vi "PH_gentec_M-Link.set i Attr.vi"(0 "i ref in":refnum<vi>, 5 "error in":errorcluster) -> (14 "i ref out":refnum<vi>, 16 "i Attributes":T1 {"Current Head Settings"."Waveform Averages" items=["None", "2", "4", "8", "16", "32", "64", "128"]; "Current Head Settings"."Trigger Source" items=["Internal", "External"]; "Current Head Settings"."Trigger Polarity" items=["Falling Edge", "Rising Edge"]; "Current Head Settings"."Measurement Mode" items=["other Mode", "Energymode"]; "Wanted Head Settings"."Waveform Averages" items=["None", "2", "4", "8", "16", "32", "64", "128"]; "Wanted Head Settings"."Trigger Source" items=["Internal", "External"]; "Wanted Head Settings"."Trigger Polarity" items=["Falling Edge", "Rising Edge"]; "Wanted Head Settings"."Measurement Mode" items=["other Mode", "Energymode"]}, 19 "error out":errorcluster)   [LabVIEW 2014, in "PH_gentec_M-Link.lvlib"]
doc: "This VI reads the DB entries and sets several attributes and GUI element settings."
uses:
  PH_gentec_M-Link.lvlib
  PH_gentec_M-Link.i attribute.ctl
  PH_gentec_M-Link.Head Settings.ctl
  instr.lib/Gentec-M-Link/Driver/Type Defs/gentec-M-Link.Measurement Mode.ctl
  instr.lib/Gentec-M-Link/Driver/Type Defs/gentec-M-Link.Trigger Polarity.ctl
  instr.lib/Gentec-M-Link/Driver/Type Defs/gentec-M-Link.Trigger Source.ctl
  instr.lib/Gentec-M-Link/Driver/Type Defs/gentec-M-Link.Waveform Averages.ctl
  instr.lib/Gentec-M-Link/gentec-M-Link - Driver.lvlib
  PH_Basics/PH_Common/PH_Common.lvlib
  CS_Core/CSSystem/CSSystemLib/CSSystemLib.lvlib
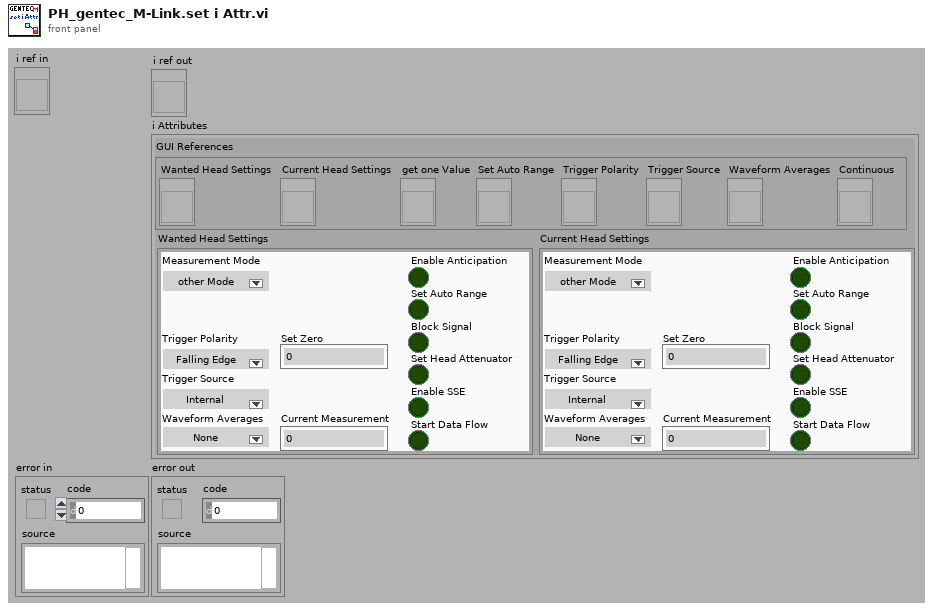
[diagram p1: front panel]
types:
  T1 = typedef "PH_gentec_M-Link.lvlib/PH_gentec_M-Link.i attribute.ctl" = cluster{"GUI References":cluster{"Wanted Head Settings":refnum<vi>, "Current Head Settings":refnum<vi>, "Set Auto Range":refnum<vi>, "Trigger Polarity":refnum<vi>, "Trigger Source":refnum<vi>, "Waveform Averages":refnum<vi>, "Continuous":refnum<vi>, "get one Value":refnum<vi>}, "Wanted Head Settings":T2, "Current Head Settings":T2}
  T2 = typedef "PH_gentec_M-Link.lvlib/PH_gentec_M-Link.Head Settings.ctl" = cluster{"Measurement Mode":T3, "Enable Anticipation":bool, "Set Auto Range":bool, "Block Signal":bool, "Set Head Attenuator":bool, "Enable SSE":bool, "Trigger Polarity":T4, "Trigger Source":T5, "Waveform Averages":T6, "Set Zero":i32, "Current Measurement":i32, "Start Data Flow":bool}
  T3 = typedef "gentec-M-Link - Driver.lvlib/gentec-M-Link.Measurement Mode.ctl" = u16
  T4 = typedef "gentec-M-Link - Driver.lvlib/gentec-M-Link.Trigger Polarity.ctl" = u16
  T5 = typedef "gentec-M-Link - Driver.lvlib/gentec-M-Link.Trigger Source.ctl" = u16
  T6 = typedef "gentec-M-Link - Driver.lvlib/gentec-M-Link.Waveform Averages.ctl" = u16
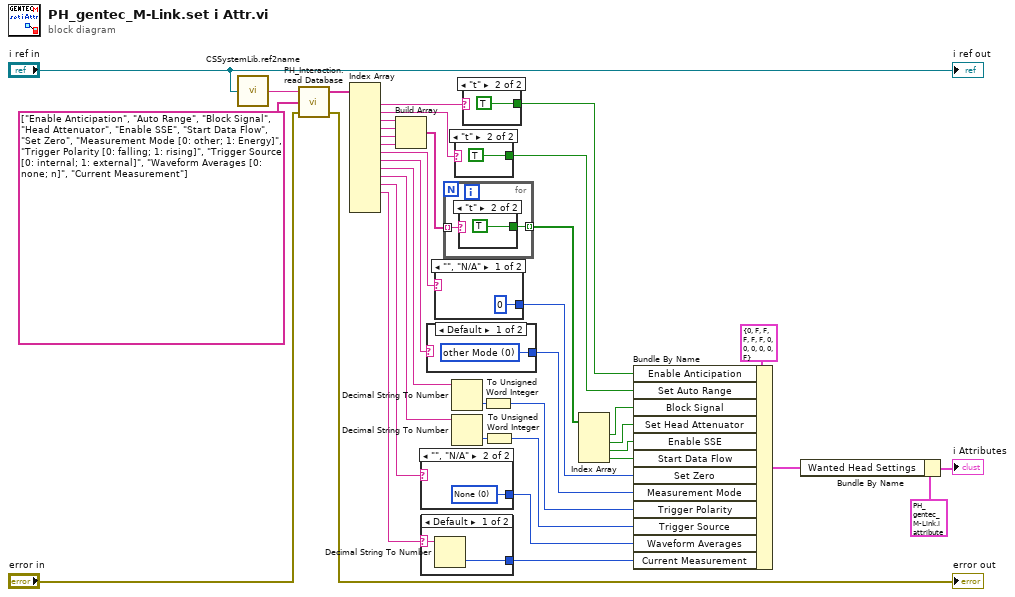
[diagram p0: block diagram]
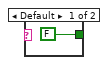
[diagram p2: hidden frame]
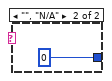
[diagram p3: hidden frame]
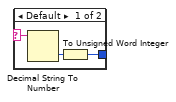
[diagram p4: hidden frame]
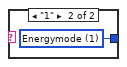
[diagram p5: hidden frame]
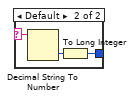
[diagram p6: hidden frame]
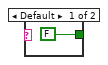
[diagram p7: hidden frame]
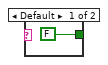
[diagram p8: hidden frame]
diagram:
  n1 = call "CSSystemLib.ref2name.vi"("obj refnum"="i ref in") -> ("name"=w19:string)
  n2 = call "PH_Interaction.read Database.vi"("error in (no error)"="error in", "Strings to search for"=string[] ["Enable Anticipation", "Auto Range", "Block Signal", "Head Attenuator", "Enable SSE", "Start Data Flow", "Set Zero", "Measurement Mode [0: other; 1: Energy]", "Trigger Polarity [0: falling; 1: rising]", "Trigger Source [0: internal; 1: external]", "Waveform Averages [0: none; n]", "Current Measurement"], "DB Entry to read"=w19) -> ("error out"=→"error out":errorcluster, "Values"=w17:string[])  [unwired: 1 in]
  n3 = Index Array(array=w17) -> (element #1=w12:string, element #2=w11:string, element #3=w10:string, element #4=w9:string, element #5=w8:string, element #6=w7:string, element #7=w6:string, element #8=w5:string, element #9=w4:string, element #10=w3:string, element #11=w2:string, element #12=w1:string)  [unwired: 14 in, 2 out]
  n4 = Build Array(w10, w9, w8, w7) -> (w33:string[])
  n5 = case shown="\"\", \"N/A\"" w2 {
    selector: w2 -> [w39 _]
    tunnel: [w40 w42] -> w24
    frame Default {
      n6 = Decimal String To Number(string=w39) -> (number=w41:i32)  [unwired: 2 in, 1 out]
      n7 = To Unsigned Word Integer(number=w41) -> (unsigned 16bit integer=w40:u16)
    }
    frame "", "N/A" {
      w42 = T6 0 items=["None", "2", "4", "8", "16", "32", "64", "128"] ("Waveform Averages")
    }
  }
  n8 = case shown="Default" w1 {
    selector: w1 -> [w44 _]
    tunnel: [w43 0 ("Current Measurement")] -> w23
    frame Default {
      n9 = Decimal String To Number(string=w44) -> (number=w43:i32)  [unwired: 2 in, 1 out]
    }
    frame "", "N/A" {
    }
  }
  n10 = case shown="Default" w5 {
    tunnel: [w46 w47] -> w36
    frame Default {
      w46 = T3 0 items=["other Mode", "Energymode"] ("Measurement Mode")
    }
    frame "1" {
      w47 = T3 1 items=["other Mode", "Energymode"] ("Measurement Mode")
    }
  }
  n11 = case shown="\"\", \"N/A\"" w6 {
    selector: w6 -> [_ w49]
    tunnel: [0 w50] -> w27
    frame "", "N/A" {
    }
    frame Default {
      n12 = Decimal String To Number(string=w49) -> (number=w51:i32)  [unwired: 2 in, 1 out]
      n13 = To Long Integer(number=w51) -> (32bit integer=w50:i32)
    }
  }
  n14 = for {
    tunnel: w33 -> [w53] mode=indexing
    tunnel: [w52] -> w32 mode=indexing
    n15 = case shown="\"t\"" w53 {
      tunnel: [FALSE ("Enable Anticipation") TRUE] -> w52
      frame Default {
      }
      frame "t" {
      }
    }
  }
  n16 = Decimal String To Number(string=w4) -> (number=w16:i32)  [unwired: 2 in, 1 out]
  n17 = Decimal String To Number(string=w3) -> (number=w15:i32)  [unwired: 2 in, 1 out]
  n18 = case shown="\"t\"" w11 {
    tunnel: [FALSE ("Enable Anticipation") TRUE] -> w34
    frame Default {
    }
    frame "t" {
    }
  }
  n19 = case shown="\"t\"" w12 {
    tunnel: [FALSE ("Enable Anticipation") TRUE] -> w35
    frame Default {
    }
    frame "t" {
    }
  }
  n20 = To Unsigned Word Integer(number=w16) -> (unsigned 16bit integer=w26:u16)
  n21 = To Unsigned Word Integer(number=w15) -> (unsigned 16bit integer=w25:u16)
  n22 = Index Array(array=w32) -> (element #1=w31:bool, element #2=w30:bool, element #3=w29:bool, element #4=w28:bool)  [unwired: 4 in]
  n23 = Bundle By Name(cluster=T2 {"Measurement Mode"=0, "Enable Anticipation"=FALSE, "Set Auto Range"=FALSE, "Block Signal"=FALSE, "Set Head Attenuator"=FALSE, "Enable SSE"=FALSE, "Trigger Polarity"=0, "Trigger Source"=0, "Waveform Averages"=0, "Set Zero"=0, "Current Measurement"=0, "Start Data Flow"=FALSE} ("Head Settings Dummy"), "Enable Anticipation"=w35, "Set Auto Range"=w34, "Block Signal"=w31, "Set Head Attenuator"=w30, "Enable SSE"=w29, "Start Data Flow"=w28, "Set Zero"=w27, "Measurement Mode"=w36, "Trigger Polarity"=w26, "Trigger Source"=w25, "Waveform Averages"=w24, "Current Measurement"=w23) -> (w21:T2)
  n24 = Bundle By Name(cluster=T1 {"GUI References"={"Wanted Head Settings"=refnum, "Current Head Settings"=refnum, "Set Auto Range"=refnum, "Trigger Polarity"=refnum, "Trigger Source"=refnum, "Waveform Averages"=refnum, "Continuous"=refnum, "get one Value"=refnum}, "Wanted Head Settings"={"Measurement Mode"=0, "Enable Anticipation"=FALSE, "Set Auto Range"=FALSE, "Block Signal"=FALSE, "Set Head Attenuator"=FALSE, "Enable SSE"=FALSE, "Trigger Polarity"=0, "Trigger Source"=0, "Waveform Averages"=0, "Set Zero"=0, "Current Measurement"=0, "Start Data Flow"=FALSE}, "Current Head Settings"={"Measurement Mode"=0, "Enable Anticipation"=FALSE, "Set Auto Range"=FALSE, "Block Signal"=FALSE, "Set Head Attenuator"=FALSE, "Enable SSE"=FALSE, "Trigger Polarity"=0, "Trigger Source"=0, "Waveform Averages"=0, "Set Zero"=0, "Current Measurement"=0, "Start Data Flow"=FALSE}} ("CLASS.i attribute"), "Wanted Head Settings"=w21) -> (→"i Attributes":T1)
  "i ref out" <- "i ref in"
